vi "Copy Buffer to Image (Default Stride ARGB).vi"(7 "Image Size":T1, 8 "error in (no error)":errorcluster, 10 "ARGB Image Destination in":T2, 11 "Buffer":u8[](array[numeric])) -> (0 "error out":errorcluster, 3 "ARGB Image Destination":T2)   [LabVIEW 2020, in "image.lvlib"]
doc: "Copy the Buffer into the Image Destination.\n\nThe Destination will be resized to acommodate the Buffer's data."
uses:
  image.lvlib
  ARGB Image.ctl
  common/Image Size (Integer).ctl
  Buffer Information.ctl
  Raw Memory Information Dimension.ctl
  f11fe23a-4bac-4ce6-b593-80dfc143e0fd.vi
  <vilib>/Utility/error.llb/Error Cluster From Error Code.vi
  common/common.lvlib
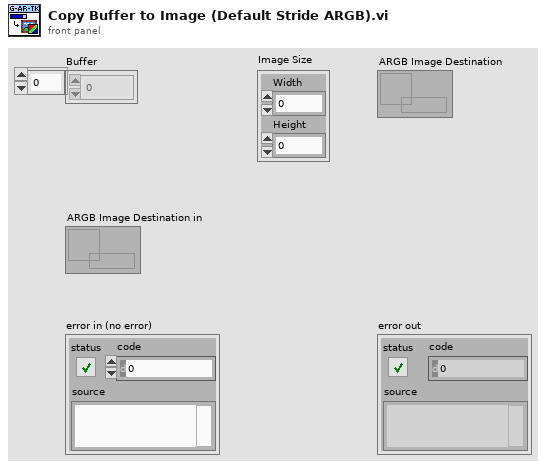
[diagram p1: front panel]
types:
  T1 = typedef "common.lvlib/Image Size (Integer).ctl" = cluster{"Width":u16, "Height":u16}
  T2 = typedef "image.lvlib/ARGB Image.ctl" = refnum<data-value>
  T3 = typedef "image.lvlib/Buffer Information.ctl" = cluster{"Dimension 0":T4, "Dimension 1":T4}
  T4 = typedef "image.lvlib/Raw Memory Information Dimension.ctl" = cluster{"Size":u16, "Stride":i32}
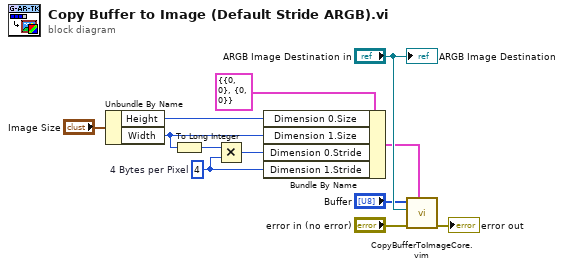
[diagram p0: block diagram]
diagram:
  w3 = 4  # 4 Bytes per Pixel
  n1 = Unbundle By Name("Image Size") -> ("Height"=w5:u16, "Width"=w4:u16)
  n2 = To Long Integer(number=w4) -> (32bit integer=w1:i32)
  n3 = Multiply(x=w1, y=w3) -> (x*y=w2:i32)
  n4 = Bundle By Name(cluster=T3 {"Dimension 0"={"Size"=0, "Stride"=0}, "Dimension 1"={"Size"=0, "Stride"=0}} ("Buffer Information"), "Dimension 0.Size"=w5, "Dimension 1.Size"=w4, "Dimension 0.Stride"=w2, "Dimension 1.Stride"=w3) -> (w7:T3)
  n5 = call "CopyBufferToImageCore.vim"("Buffer Information"=w7, "error in (no error)"="error in (no error)", "Dst"="ARGB Image Destination in", "Buffer"="Buffer") -> ("error out"=→"error out":errorcluster)  [unwired: 7 in]
  "ARGB Image Destination" <- "ARGB Image Destination in"
